vi "SHA-1 (String).vi"(10 "message":string) -> (2 "SHA-1 hash":string)   [LabVIEW 2013, in "SHA-1.lvlib"]
uses:
  SHA-1.lvlib
  SHA-1.lvclass
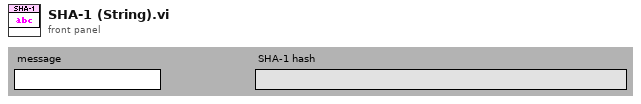
[diagram p1: front panel]
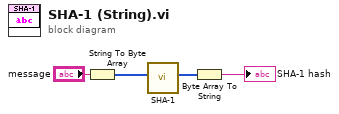
[diagram p0: block diagram]
diagram:
  n1 = String To Byte Array(string="message") -> (unsigned byte array=w2:u8[])
  n2 = call "SHA-1.vi"("data"=w2) -> ("SHA-1 hash"=w3:u8[])  [unwired: 10 in]
  n3 = Byte Array To String(unsigned byte array=w3) -> (string=→"SHA-1 hash":string)
